vi "SPD.DCR Meas.vi"(5 "Continue":refnum<vi>, 7 "Progress":refnum<vi>, 8 "Error In":errorcluster, 10 "DCRParams":T1, 11 "SPD.Stand Ctrl in":T2 {"spdDeviceSession"."hidSPD.Controller"."HV_bias" format="%#_6p, V"; "spdDeviceSession"."hidSPD.Controller"."TSet" format="%#_6p, DegC"}) -> (0 "Error Out":errorcluster, 1 "pass":bool, 2 "result":string, 3 "SPD.Stand Ctrl out":T2 {"spdDeviceSession"."hidSPD.Controller"."HV_bias" format="%#_6p, V"; "spdDeviceSession"."hidSPD.Controller"."TSet" format="%#_6p, DegC"})   [LabVIEW 2018]
uses:
  typedefs/SPD.Stand Ctrl.ctl
  Instruments/SPD HID Interface/hidSPDLibForLabView/LibVIs/hidSPD Controls/hidSPD Device Session.ctl
  Instruments/SPD HID Interface/hidSPDLibForLabView/LibVIs/hidSPD Controls/hidSPD Controller.ctl
  Instruments/KC705 DevBoard/typedefs/DevB.Session.ctl
  Instruments/KeySight 53230A/typedefs/FreqC.Session.ctl
  Instruments/KeySight 8164B/KeySight 8164B LAN InstrLib/typedefs/KeySight 8164B control.ctl
  Instruments/LeCroy SDA830/typedefs/LeCroy.Session.ctl
  typedefs/SPD.Events.ctl
  <vilib>/Utility/config.llb/Config Data RefNum.ctl
  typedefs/SPD.Meas Result.ctl
  SPD.DCR Test Params.ctl
  Instruments/KeySight 8164B/KeySight 8164B LAN InstrLib.lvlib
  Instruments/SPD HID Interface/hidSPDLibForLabView/hidSPDLibForLabView.lvlib
  <vilib>/Utility/config.llb/NI_LVConfig.lvlib
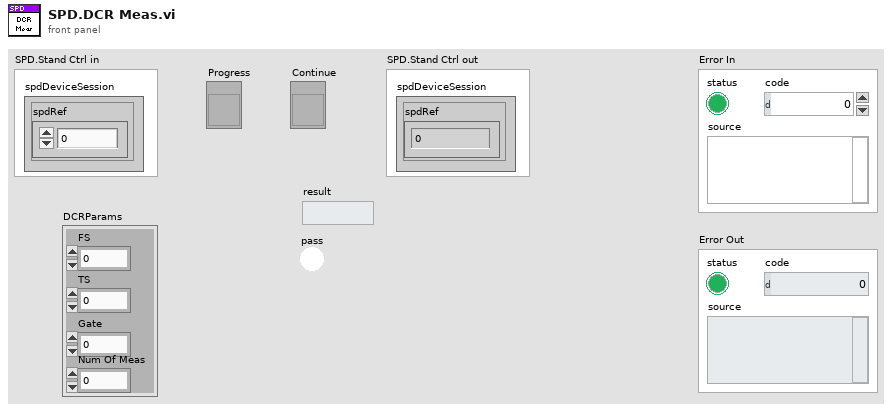
[diagram p1: front panel]
types:
  T1 = typedef "SPD.DCR Test Params.ctl" = cluster{"FS":i32, "TS":i32, "Gate":dbl, "Num Of Meas":i32}
  T2 = typedef "SPD.Stand Ctrl.ctl" = cluster{"spdDeviceSession":T3, "DevBSession":T5, "FreqCSession":T6, "8164BSession":T7, "LeCroySession":T8, "Events":T9, "configFile":T10, "SPD.Result":T11}
  T3 = typedef "hidSPDLibForLabView.lvlib/hidSPD Device Session.ctl" = cluster{"spdRef":u64, "connected":bool, "spdName":string, "hidSPD.Controller":T4}
  T4 = typedef "hidSPDLibForLabView.lvlib/hidSPD Controller.ctl" = cluster{"TSet":sgl, "HV_bias":sgl, "DDS_stb_code":u16}
  T5 = typedef "DevB.Session.ctl" = cluster{"DevBRef":refnum<visa-resource-name>, "connected":bool}
  T6 = typedef "FreqC.Session.ctl" = cluster{"FreqCRef":refnum<visa-resource-name>, "timeout":dbl, "Gate":dbl, "connected":bool}
  T7 = typedef "KeySight 8164B LAN InstrLib.lvlib/KeySight 8164B control.ctl" = cluster{"Connection ID":refnum<k5>, "Connected":bool, "Info":string, "Slots Info":string[]}
  T8 = typedef "LeCroy.Session.ctl" = cluster{"LeCroySession":refnum<visa-resource-name>, "connected":bool}
  T9 = typedef "SPD.Events.ctl" = cluster{"DCRTest":refnum<user-event>, "Stop":refnum<user-event>}
  T10 = typedef "NI_LVConfig.lvlib/Config Data RefNum.ctl" = refnum<k1>
  T11 = typedef "SPD.Meas Result.ctl" = cluster{"HV_Bias":dbl[][][], "Stb_code":dbl[], "Temprature":dbl[], "Data":dbl[][][][]}
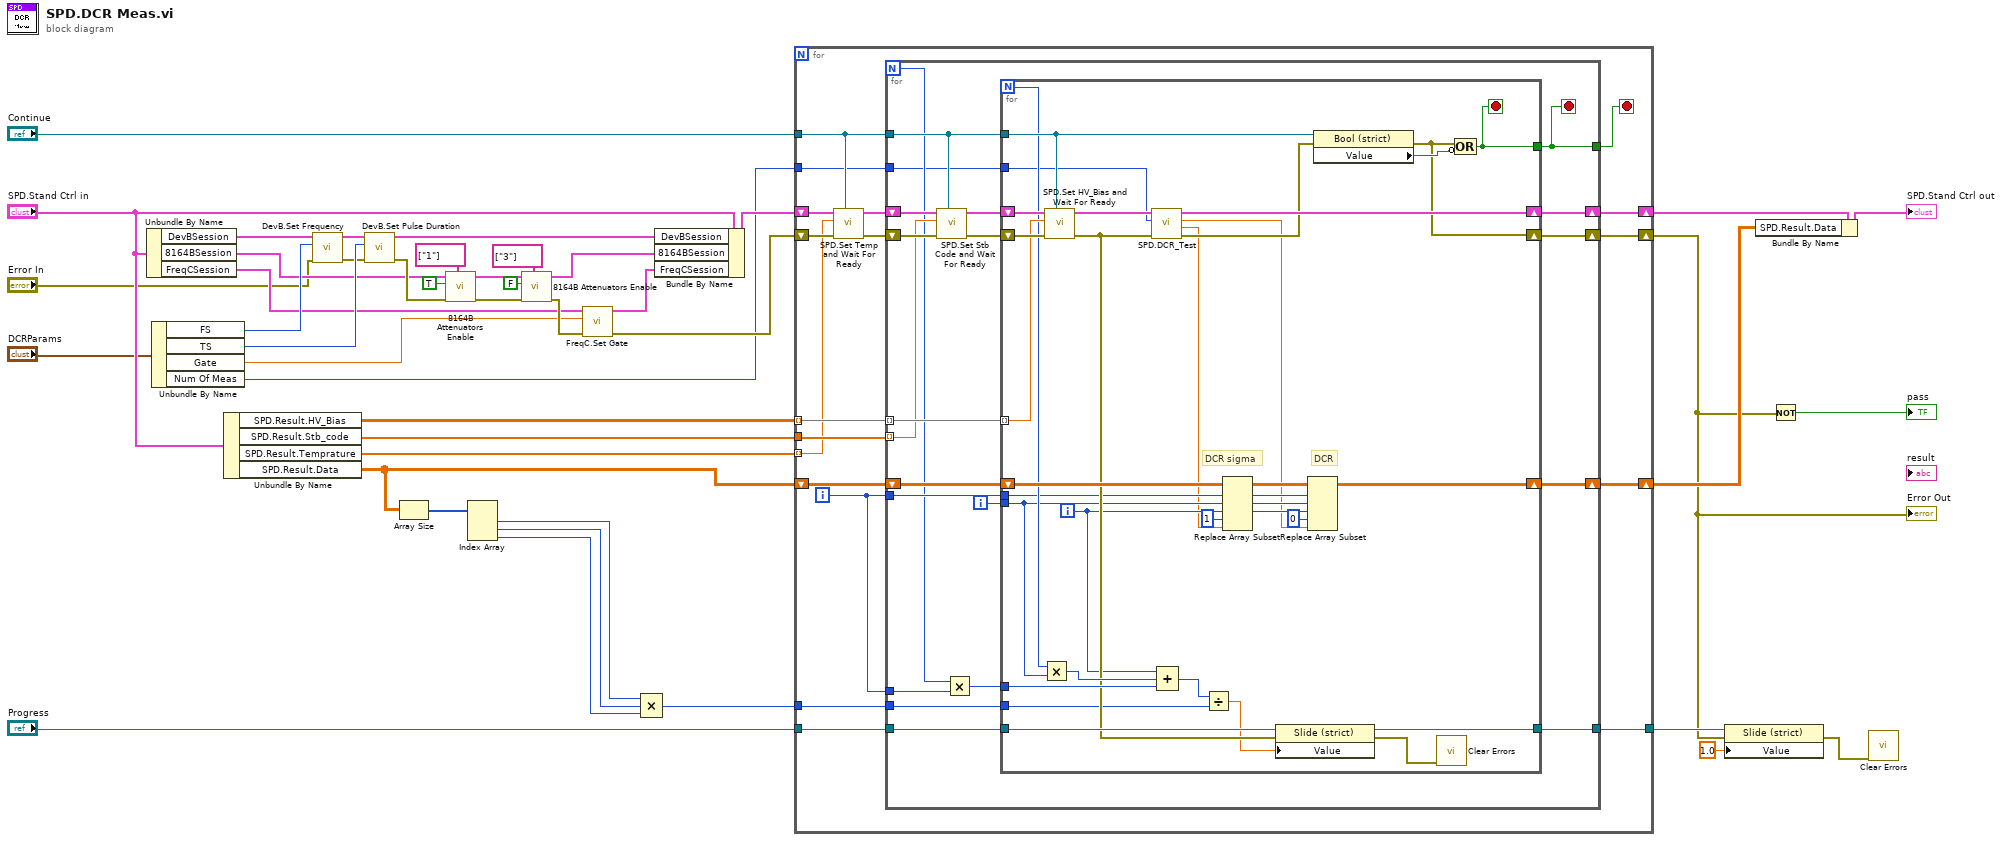
[diagram p0: block diagram]
diagram:
  n1 = Unbundle By Name("SPD.Stand Ctrl in") -> ("DevBSession"=w30:T5, "8164BSession"=w17:T7, "FreqCSession"=w16:T6)
  n2 = Unbundle By Name("DCRParams") -> ("FS"=w28:i32, "TS"=w27:i32, "Gate"=w9:dbl, "Num Of Meas"=w6:i32)
  n3 = Unbundle By Name("SPD.Stand Ctrl in") -> ("SPD.Result.HV_Bias"=w31:dbl[][][], "SPD.Result.Stb_code"=w32:dbl[], "SPD.Result.Temprature"=w33:dbl[], "SPD.Result.Data"=w5:dbl[][][][])
  n4 = call "DevB.Set Frequency.vi"("error in (no error)"="Error In", "Frequency"=w28, "DevB Session in"=w30) -> ("error out"=w26:errorcluster, "DevB Session out"=w29:T5)  [unwired: 7 in]
  n5 = call "DevB.Set Pulse Duration.vi"("error in (no error)"=w26, "Pulse Duration"=w27, "DevB Session in"=w29) -> ("error out"=w19:errorcluster, "DevB Session out"=w15:T5)  [unwired: 7 in]
  n6 = Array Size(array=w5) -> (size(s)=w4:i32[])
  n7 = call "8164B Attenuators Enable.vi"("Slots"=string[] ["1"], "error in"=w19, "Enable"=TRUE, "KeySight 8164B control in"=w17) -> ("error out"=w23:errorcluster, "KeySight 8164B control out"=w22:T7)  [unwired: 6 in]
  n8 = Index Array(array=w4) -> (element #1=w3:i32, element #2=w2:i32, element #3=w1:i32)  [unwired: 3 in]
  n9 = call "8164B Attenuators Enable.vi"("Slots"=string[] ["3"], "error in"=w23, "Enable"=FALSE, "KeySight 8164B control in"=w22) -> ("error out"=w18:errorcluster, "KeySight 8164B control out"=w14:T7)  [unwired: 6 in]
  n10 = call "FreqC.Set Gate.vi"("error In"=w18, "Gate, sec"=w9, "FreqC Session in"=w16) -> ("error out"=w10:errorcluster, "FreqC Session out"=w13:T6)  [unwired: 7 in]
  n11 = Compound Arithmetic op=MULTIPLY(w3, w2, w1) -> (w38:i32)
  n12 = Bundle By Name(cluster="SPD.Stand Ctrl in", "DevBSession"=w15, "8164BSession"=w14, "FreqCSession"=w13) -> (w11:T2)
  n13 = for {
    shift-right: [w58] -> w41
    shift-left: w5 -> [w62]
    tunnel: w31 -> [w61] mode=indexing
    shift-right: [w60] -> w44
    shift-left: w11 -> [w56]
    tunnel: w32 -> [w59]
    tunnel: w33 -> [w53] mode=indexing
    shift-right: [w57] -> w34
    shift-left: w10 -> [w55]
    tunnel: "Continue" -> [w51]
    tunnel: "Progress" -> [w48]
    tunnel: w38 -> [w47]
    tunnel: [w46] -> w37
    tunnel: w6 -> [w45]
    i -> [w49]
    stop <- w50 stop-if-true
    n14 = call "SPD.Set Temp and Wait For Ready.vi"("Continue"=w51, "Error In"=w55, "Tset"=w53, "SPD.Stand Ctrl in"=w56) -> ("Error Out"=w54:errorcluster, "SPD.Stand Ctrl out"=w52:T2)  [unwired: 6 in]
    n15 = for {
      N -> [w68]
      shift-right: [w80] -> w58
      shift-left: w62 -> [w82]
      tunnel: w61 -> [w83] mode=indexing
      tunnel: w59 -> [w74] mode=indexing
      shift-right: [w81] -> w60
      shift-left: w52 -> [w78]
      shift-right: [w79] -> w57
      shift-left: w54 -> [w76]
      tunnel: w51 -> [w73]
      tunnel: w49 -> [w72]
      tunnel: [w70] -> w50
      tunnel: w49 -> [w69]
      tunnel: w48 -> [w66]
      tunnel: w47 -> [w65]
      tunnel: [w64] -> w46
      tunnel: w45 -> [w63]
      i -> [w71]
      stop <- w70 stop-if-true
      n16 = call "SPD.Set Stb Code and Wait For Ready.vi"("Continue"=w73, "Error In"=w76, "Strobe code"=w74, "SPD.Stand Ctrl in"=w78) -> ("Error Out"=w75:errorcluster, "SPD.Stand Ctrl out"=w77:T2)  [unwired: 6 in]
      n17 = Multiply(x=w68, y=w69) -> (x*y=w67:i32)
      n18 = for {
        N -> [w103]
        tunnel: w83 -> [w108] mode=indexing
        shift-right: [w91] -> w80
        shift-left: w82 -> [w114]
        shift-right: [w113] -> w81
        shift-left: w77 -> [w111]
        shift-right: [w105] -> w79
        shift-left: w75 -> [w109]
        tunnel: w73 -> [w107]
        tunnel: w72 -> [w90]
        tunnel: w71 -> [w89]
        tunnel: [w104] -> w70
        tunnel: w67 -> [w101]
        tunnel: w66 -> [w100]
        tunnel: w65 -> [w97]
        tunnel: [w95] -> w64
        tunnel: w63 -> [w84]
        i -> [w88]
        stop <- w104 stop-if-true
        # "DCR"
        # "DCR sigma"
        n19 = Multiply(x=w103, y=w89) -> (x*y=w102:i32)
        n20 = call "SPD.Set HV_Bias and Wait For Ready.vi"("Continue"=w107, "Error In"=w109, "HV_Bias"=w108, "SPD.Stand Ctrl in"=w111) -> ("Error Out"=w99:errorcluster, "SPD.Stand Ctrl out"=w110:T2)  [unwired: 6 in]
        n21 = call "SPD.DCR_Test.vi"("Error In"=w99, "Num of Meas"=w84, "SPD.Stand Ctrl in"=w110) -> ("Error Out"=w112:errorcluster, "DCR sigma"=w86:dbl, "DCR"=w85:dbl, "SPD.Stand Ctrl out"=w113:T2)  [unwired: 5 in]
        n22 = Compound Arithmetic op=ADD(w88, w102, w101) -> (w98:i32)
        n23 = Divide(x=w98, y=w97) -> (x/y=w96:dbl)
        n24 = Replace Array Subset(array=w114, new element=w86, index (dim 0)=w90, index (dim 1)=w89, index (dim 2)=w88, index (dim 3)=1 ("disabled index (col)")) -> (w92:dbl[][][][])
        n25 = property class="Slide (strict)"(reference=w100, error in=w99, "Value"=w96) -> (reference out=w95:refnum<vi>, error out=w94:errorcluster)
        n26 = Replace Array Subset(array=w92, new element=w85, index (dim 0)=w90, index (dim 1)=w89, index (dim 2)=w88, index (dim 3)=0 ("disabled index (col)")) -> (w91:dbl[][][][])
        n27 = property class="Bool (strict)"(reference=w107, error in=w112) -> (error out=w105:errorcluster, "Value"=w106:bool)  [unwired: 1 out]
        n28 = call <vilib>:"Clear Errors.vi"("error in (no error)"=w94) -> ()  [unwired: 5 in, 2 out]
        n29 = Compound Arithmetic op=OR(w105, invert w106) -> (w104:bool)
      }
    }
  }
  "Error Out" <- w34
  n30 = property class="Slide (strict)"(reference=w37, error in=w34, "Value"=1.0) -> (error out=w35:errorcluster)  [unwired: 1 out]
  n31 = Bundle By Name(cluster=w44, "SPD.Result.Data"=w41) -> (→"SPD.Stand Ctrl out":T2)
  n32 = Not(x=w34) -> (.not. x?=→"pass":bool)
  n33 = call <vilib>:"Clear Errors.vi"("error in (no error)"=w35) -> ()  [unwired: 5 in, 2 out]
